vi "EXDIR-YAML_CountSpaces.vi"(11 "String":string) -> (3 "Numeric":i32)   [LabVIEW 2016]
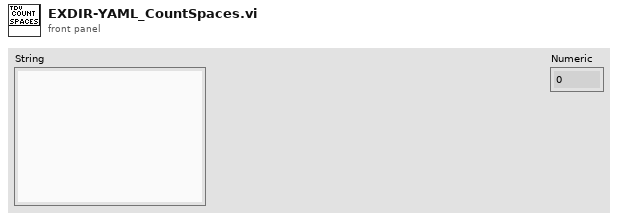
[diagram p1: front panel]
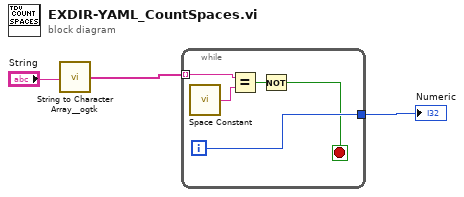
[diagram p0: block diagram]
diagram:
  n1 = call <userlib>:"String to Character Array__ogtk.vi"("Input String"="String") -> ("Character Array"=w1:string[])
  n2 = while {
    tunnel: w1 -> [w8] mode=indexing
    tunnel: [w7] -> w2
    i -> [w7]
    stop <- w5 stop-if-true
    n3 = call <vilib>:"Space Constant.vi"() -> ("String"=w4:string)
    n4 = Equal?(x=w8, y=w4) -> (x = y?=w6:bool)
    n5 = Not(x=w6) -> (.not. x?=w5:bool)
  }
  "Numeric" <- w2
